vi "GetWaveformOrderByName.vi"(8 "error in (no error)":errorcluster, 10 "Channel Name":string, 11 "Acq Waveforms":waveform(sgl)[](array[waveform])) -> (0 "error out":errorcluster, 1 "Waveform Channel Order":i32, 2 "Found?":bool, 3 "Acq Waveforms Out":waveform(sgl)[](array[waveform]))   [LabVIEW 2017, in "McsaUtilities.lvlib"]
uses:
  <vilib>/addons/InsightCM/Utilities/MCSA/McsaUtilities.lvlib
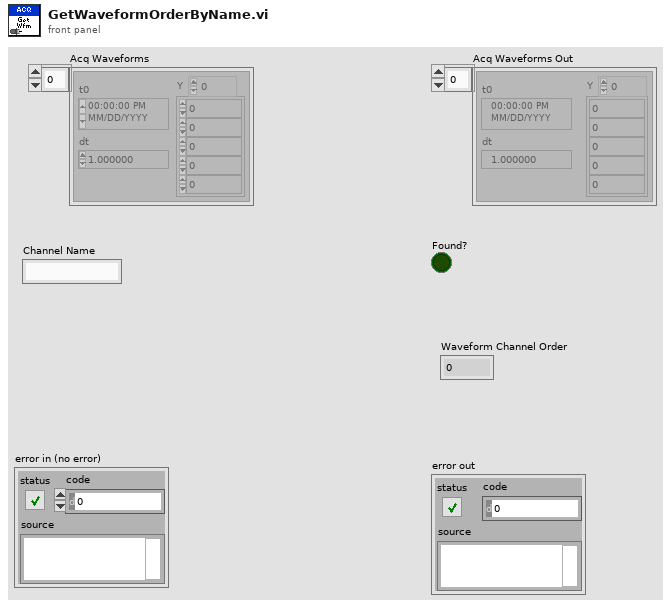
[diagram p1: front panel]
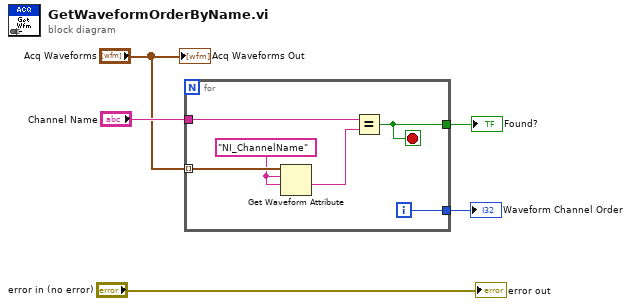
[diagram p0: block diagram]
diagram:
  n1 = for {
    tunnel: "Acq Waveforms" -> [w11] mode=indexing
    tunnel: "Channel Name" -> [w10]
    tunnel: [w7] -> w3
    tunnel: [w6] -> w1
    i -> [w6]
    stop <- w7 stop-if-true
    w9 = "NI_ChannelName" ("name")
    n2 = Get Waveform Attribute(5:w9, 6:w9, 7:w11) -> (1:w8:string)  [unwired: 1 in, 3 out]
    n3 = Equal?(x=w10, y=w8) -> (x = y?=w7:bool)
  }
  "Found?" <- w3
  "Waveform Channel Order" <- w1
  "Acq Waveforms Out" <- "Acq Waveforms"
  "error out" <- "error in (no error)"
